vi "EmptyLog.vi"(8 "Error in (no error)":errorcluster, 11 "LogWriterMock in":refnum<class "LogWriterMock.lvclass">) -> (0 "Error out":errorcluster, 3 "LogWriterMock out":refnum<class "LogWriterMock.lvclass">)   [LabVIEW 2011, in "LogWriterMock.lvclass"]
uses:
  LogWriterMock.lvclass
  Log/LogCluster.ctl
  Log/PrioritiesRing.ctl
  LogWriterMock.lvclass/LogWriterMock.ctl
  Log/Log.lvclass
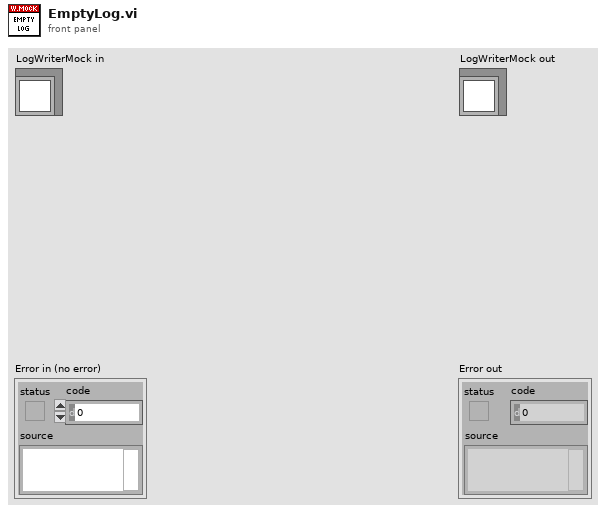
[diagram p1: front panel]
types:
  T1 = typedef "Log.lvclass/LogCluster.ctl" = cluster{"Timestamp":string, "Message":string, "Priority":T2, "PriorityName":string}
  T2 = typedef "Log.lvclass/PrioritiesRing.ctl" = u32
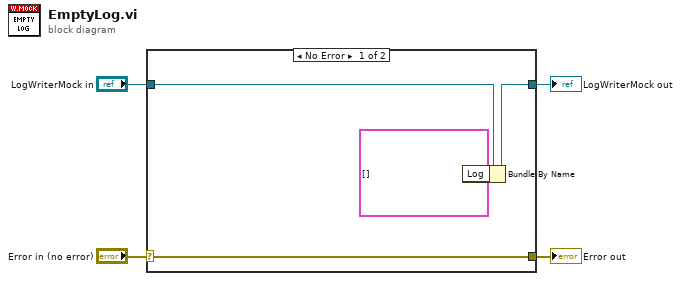
[diagram p0: block diagram]
diagram:
  n1 = case shown="No Error" "Error in (no error)" {
    selector: "Error in (no error)" -> [w8 w9]
    tunnel: [w8 w9] -> w3
    tunnel: [w6 w10] -> w1
    tunnel: "LogWriterMock in" -> [w7 w10]
    frame No Error {
      n2 = Bundle By Name(cluster=w7, "Log"=T1[] []) -> (w6:refnum<class "LogWriterMock.lvclass">)
    }
    frame Error {
    }
  }
  "Error out" <- w3
  "LogWriterMock out" <- w1
